vi "Write Status.vi"(8 "error in (no error)":errorcluster, 10 "Status":enum16{"Closed", "Open"}(ring), 11 "Solenoid Valve.lvclass in":refnum<class "Solenoid Valve.lvclass">) -> (0 "error out":errorcluster, 3 "Solenoid Valve.lvclass out":refnum<class "Solenoid Valve.lvclass">)   [LabVIEW 2011, in "Solenoid Valve.lvclass"]
uses:
  Solenoid Valve.lvclass
  Solenoid Valve.lvclass/Solenoid Valve.ctl
  <vilib>/DAQmx/write.llb/DAQmx Write (Digital Bool 1Line 1Point).vi
  <vilib>/DAQmx/miscellaneous.llb/DAQmx Fill In Error Info.vi
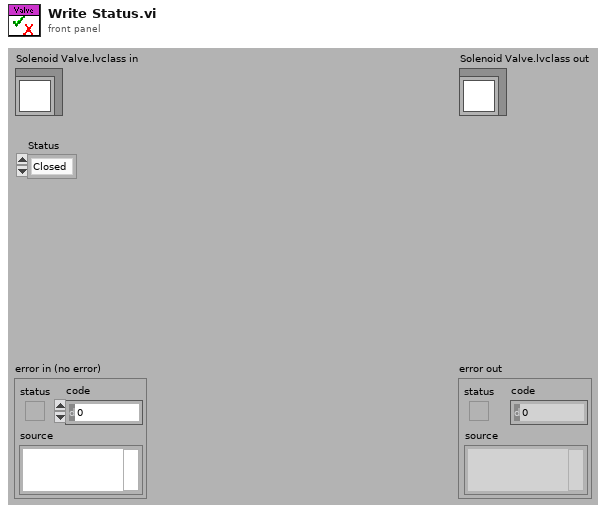
[diagram p1: front panel]
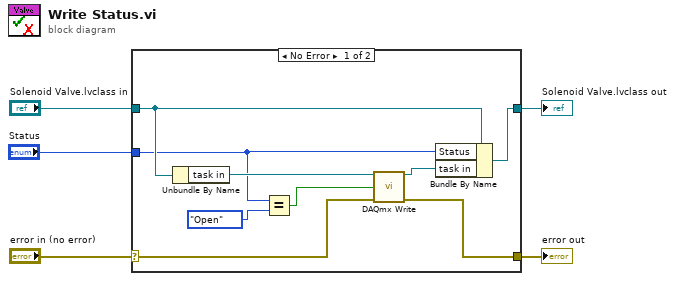
[diagram p0: block diagram]
diagram:
  n1 = case shown="No Error" "error in (no error)" {
    selector: "error in (no error)" -> [w7 w15]
    tunnel: [w6 w15] -> w4
    tunnel: [w14 w16] -> w2
    tunnel: "Solenoid Valve.lvclass in" -> [w13 w16]
    tunnel: "Status" -> [w11 _]
    frame No Error {
      n2 = Unbundle By Name(w13) -> ("task in"=w12:refnum<k21>)
      n3 = Equal?(x=w11, y=enum16{"Closed", "Open"}."Open") -> (x = y?=w9:bool)
      n4 = call-poly <vilib>:"DAQmx Write.vi"("task/channels in"=w12, "data"=w9, "error in"=w7) -> ("task out"=w8:refnum<k21>, "error out"=w6:errorcluster)  [unwired: 10 in, 1 out]
      n5 = Bundle By Name(cluster=w13, "Status"=w11, "task in"=w8) -> (w14:refnum<class "Solenoid Valve.lvclass">)
    }
    frame Error {
    }
  }
  "error out" <- w4
  "Solenoid Valve.lvclass out" <- w2
